vi "Burn-In Testing.vi"() -> ()   [LabVIEW 2012]
uses:
  TestData/Command.ctl
  Controls/Command_Enum.ctl
  Controls/Exit.vi
  Controls/MainRef.ctl
  Controls/Waferimage.ctl
  Controls/TestData.ctl
  Controls/UserInput.ctl
  Controls/MeasureControl.ctl
  Controls/TestArea.ctl
  Controls/WaferDataDisplay.ctl
  Controls/MapPOS.ctl
panel:
  in  "Stop":bool
  in  "Input":T1
  in  "Calibration Wl":dbl
  in  "Wl min,nm":dbl
  in  "Wl max,nm":dbl
  in  "GPIB":string
  in  "Integration Time":i32
  in  "Stop Current,mA":dbl
  in  "Start Current,mA":dbl
  in  "Voltage Compliance,V":dbl
  in  "QuickTest_Display":T2 {"TestData"."50mA Data"."Current,mA" format="%_6g"; "TestData"."50mA Data"."WL" format="%_6g"; "TestData"."50mA Data"."Voltage" format="%_6g"; "TestData"."50mA Data"."Power" format="%_6g"; "TestData"."20mA Data"."Reverse" format="%#_3g"; "TestData"."20mA Data"."Current,mA" format="%_6g"; "TestData"."20mA Data"."Knee Current" format="%#_3g"; "TestData"."20mA Data"."WL" format="%_6g"; "TestData"."20mA Data"."Voltage" format="%_6g"; "TestData"."20mA Data"."Power" format="%_5g"}
  in  "System Back Button":bool
  in  "MapPOS":T5={"Top"={"left"=208, "top"=106, "right"=218, "bottom"=116}, "CenterC"={"left"=217, "top"=189, "right"=228, "bottom"=200}, "CenterB"={"left"=217, "top"=208, "right"=228, "bottom"=219}, "CenterA"={"left"=199, "top"=208, "right"=209, "bottom"=219}, "Left"={"left"=103, "top"=199, "right"=114, "bottom"=209}, "Right"={"left"=314, "top"=199, "right"=325, "bottom"=209}}
  in  "Wafer Data":T6
  out "Wafer":T7
  # "Current Result"
  # "Measure Control"
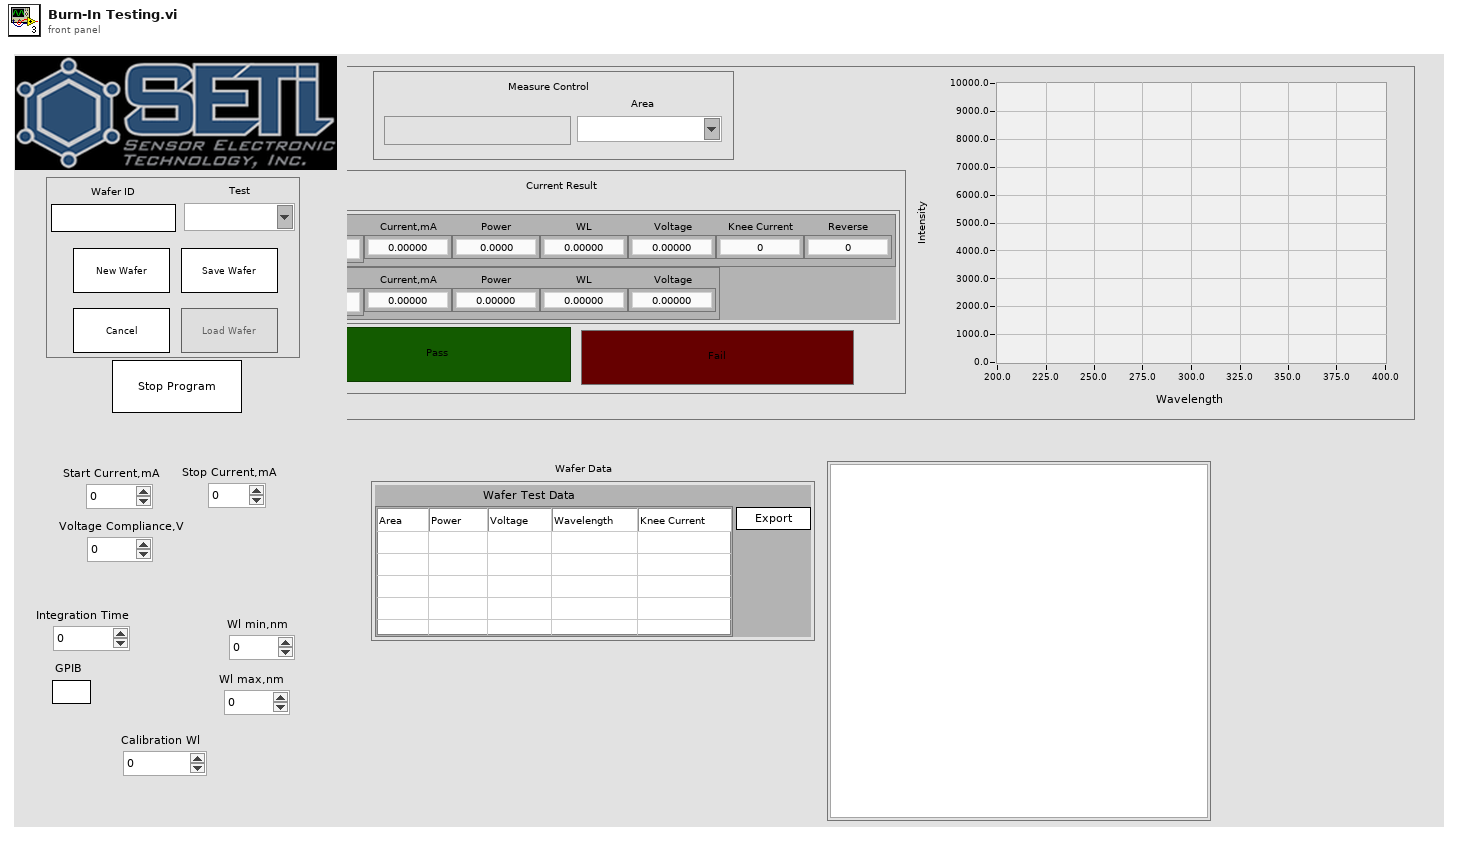
[diagram p1: front panel]
types:
  T1 = typedef "UserInput.ctl" = cluster{"Wafer ID":string, "Test":string, "New":bool, "Save":bool, "Load":bool, "Cancel":bool}
  T2 = typedef "MeasureControl.ctl" = cluster{"Pass":bool, "Fail":bool, "Measure":bool, "Area":T3, "TestData":T4, "Graph":cluster{"Y":dbl[], "Y":dbl[]}[]}
  T3 = typedef "TestArea.ctl" = string
  T4 = typedef "TestData.ctl" = cluster{"20mA Data":cluster{"Area":string, "Current,mA":dbl, "Power":dbl, "WL":dbl, "Voltage":dbl, "Knee Current":dbl, "Reverse":dbl}, "50mA Data":cluster{"Area":string, "Current,mA":dbl, "Power":dbl, "WL":dbl, "Voltage":dbl}}
  T5 = typedef "MapPOS.ctl" = cluster{"Top":cluster{"left":i16, "top":i16, "right":i16, "bottom":i16}, "CenterC":cluster{"left":i16, "top":i16, "right":i16, "bottom":i16}, "CenterB":cluster{"left":i16, "top":i16, "right":i16, "bottom":i16}, "CenterA":cluster{"left":i16, "top":i16, "right":i16, "bottom":i16}, "Left":cluster{"left":i16, "top":i16, "right":i16, "bottom":i16}, "Right":cluster{"left":i16, "top":i16, "right":i16, "bottom":i16}}
  T6 = typedef "WaferDataDisplay.ctl" = cluster{"Wafer Test Data":string[][], "Export":bool}
  T7 = typedef "Waferimage.ctl" = picture
  T8 = typedef "MainRef.ctl" = cluster{"Wafer Data":refnum<vi>, "MeasureCntrl":refnum<vi>, "Input":refnum<vi>, "Wafer":refnum<vi>, "MapPOS":refnum<vi>, "INSTR_PARAM 2":refnum<vi>}
  T9 = typedef "Command.ctl" = cluster{"Command":T10, "Data":variant, "type":variant}
  T10 = typedef "Command_Enum.ctl" = enum16{"INIT", "LOAD", "MEASURE", "NEW", "SAVE", "SWAP_MODE", "UPDATE_ACQ", "EXIT", "CANCEL"}
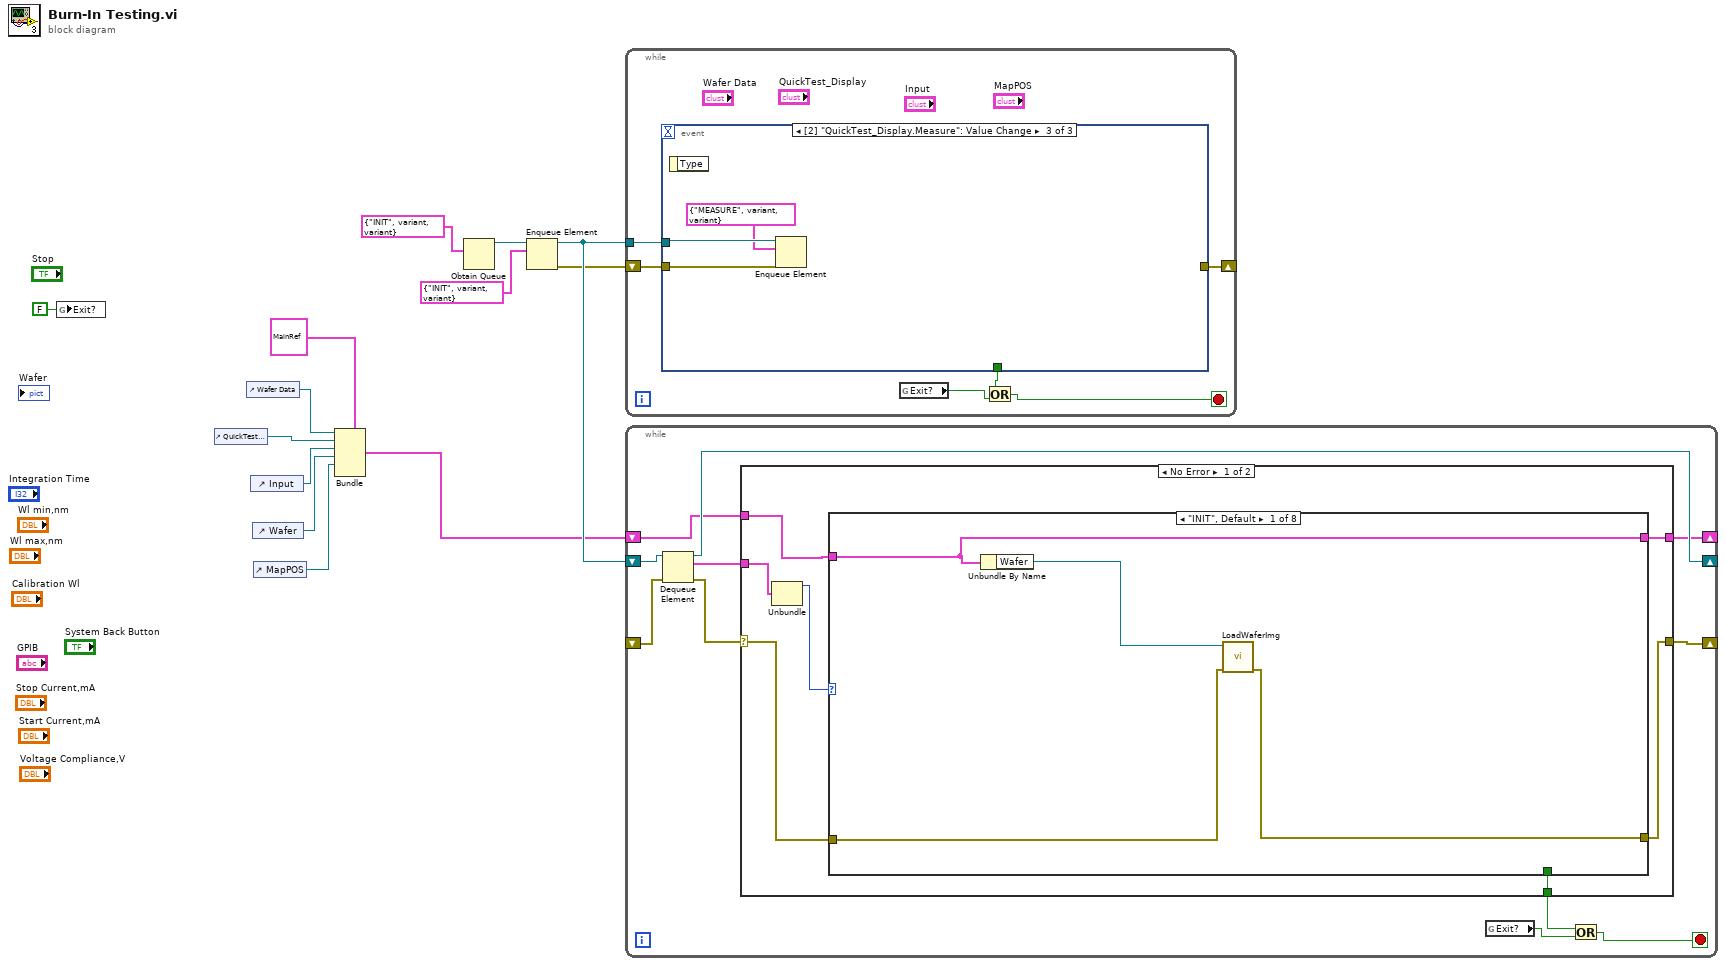
[diagram p0: block diagram]
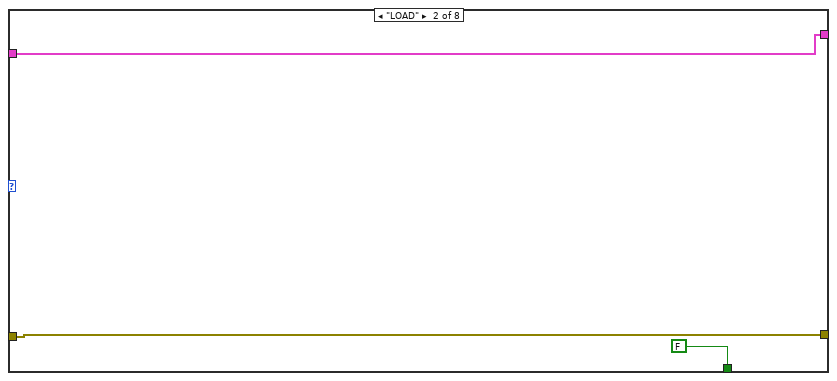
[diagram p2: hidden frame]
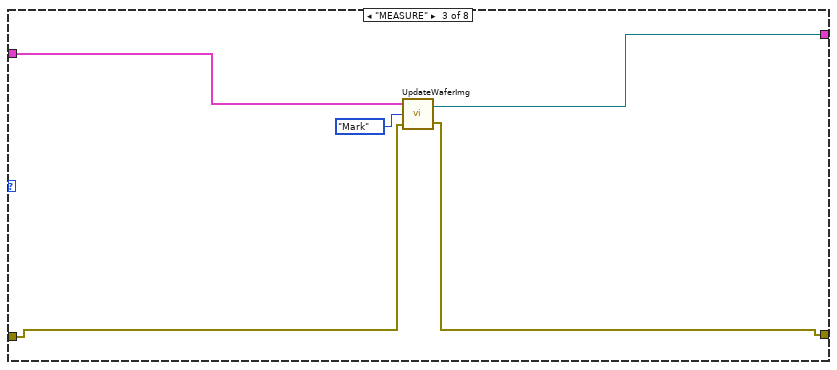
[diagram p3: hidden frame]
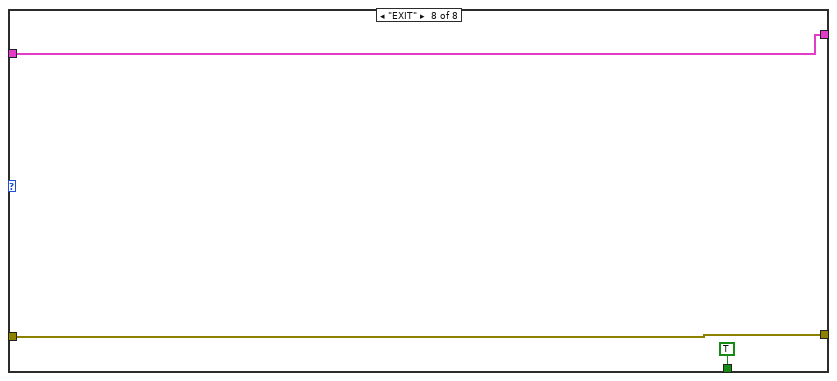
[diagram p8: hidden frame]
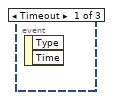
[diagram p10: hidden frame]
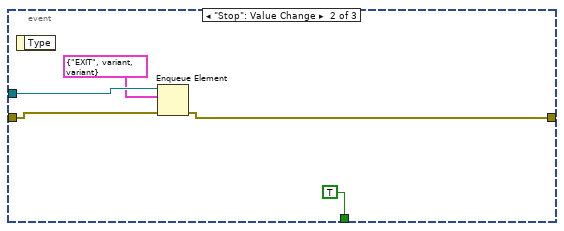
[diagram p11: hidden frame]
diagram:
  n1 = global write "Exit.vi" "Exit?"(FALSE ("Exit?")) -> ()
  n2 = control-ref of="QuickTest_Display"() -> (w6:refnum<vi>)
  n3 = control-ref of="Wafer Data"() -> (w7:refnum<vi>)
  n4 = control-ref of="Input"() -> (w5:refnum<vi>)
  n5 = control-ref of="Wafer"() -> (w4:refnum<vi>)
  n6 = control-ref of="MapPOS"() -> (w2:refnum<vi>)
  n7 = Bundle(cluster=T8 {"Wafer Data"=refnum, "MeasureCntrl"=refnum, "Input"=refnum, "Wafer"=refnum, "MapPOS"=refnum, "INSTR_PARAM 2"=refnum}, "Wafer Data"=w7, "MeasureCntrl"=w6, "Input"=w5, "Wafer"=w4, "MapPOS"=w2) -> (w3:T8)  [unwired: 1 in]
  n8 = Obtain Queue(element data type=T9 {"Command"=enum."INIT", "Data"=variant, "type"=variant} ("Cluster")) -> (queue out=w12:refnum<queue>)  [unwired: 4 in, 2 out]
  n9 = Enqueue Element(queue=w12, element=T9 {"Command"=enum."INIT", "Data"=variant, "type"=variant}) -> (queue out=w10:refnum<queue>, error out=w9:errorcluster)  [unwired: 2 in, 1 out]
  n10 = while {
    tunnel: w10 -> [w19]
    shift-right: [w14] -> _
    shift-left: w9 -> [w15]
    stop <- w17 stop-if-true
    n11 = event shown="[2] \"QuickTest_Display.Measure\": Value Change" {
      selector: _ -> [_ _ _]
      dyn-events: _ -> [_ _ _]
      timeout: _ -> [_ _ _]
      tunnel: w19 -> [_ w23 w27]
      tunnel: [_ TRUE ("x") _] -> w16
      tunnel: w15 -> [_ w21 w26]
      tunnel: [_ w20 _] -> w14
      event Timeout {
        n12 = event-data() -> ()  [unwired: 1 in, 2 out]
      }
      event "Stop": Value Change {
        n13 = event-data() -> ()  [unwired: 1 in, 1 out]
        n14 = Enqueue Element(queue=w23, element=T9 {"Command"=enum."EXIT", "Data"=variant, "type"=variant}, error in (no error)=w21) -> (error out=w20:errorcluster)  [unwired: 1 in, 2 out]
      }
      event Value Change {
        n15 = event-data() -> ()  [unwired: 1 in, 1 out]
        n16 = Enqueue Element(queue=w27, element=T9 {"Command"=enum."MEASURE", "Data"=variant, "type"=variant}, error in (no error)=w26) -> ()  [unwired: 1 in, 3 out]
      }
    }
    n17 = global read "Exit.vi" "Exit?"() -> (w18:bool)
    n18 = Or(x=w16, y=w18) -> (x .or. y?=w17:bool)
  }
  n19 = while {
    shift-right: [w34] -> _
    shift-left: w10 -> [w38]
    shift-right: [w35] -> _
    shift-left: _ -> [w36]
    shift-right: [w28] -> _
    shift-left: w3 -> [w29]
    stop <- w31 stop-if-true
    n20 = Dequeue Element(queue=w38, error in (no error)=w36) -> (queue out=w34:refnum<queue>, element=w33:T9, error out=w37:errorcluster)  [unwired: 1 in, 1 out]
    n21 = case shown="No Error" w37 {
      selector: w37 -> [w41 w70]
      tunnel: [w42 w70] -> w35
      tunnel: w33 -> [w45 _]
      tunnel: [w43 _] -> w30
      tunnel: w29 -> [w40 w69]
      tunnel: [w39 w69] -> w28
      frame No Error {
        n22 = Unbundle(w45) -> ("Command"=w44:T10)  [unwired: 2 out]
        n23 = case shown="\"INIT\", Default" w44 {
          tunnel: [_ FALSE ("y") _ _ _ _ _ TRUE ("y")] -> w43
          tunnel: [w46 w51 w54 w59 w61 w63 w65 w67] -> w42
          tunnel: w41 -> [w49 w51 w53 w59 w61 w63 w65 w67]
          tunnel: w40 -> [w48 w50 w56 w58 w60 w62 w64 w66]
          tunnel: [w48 w50 w55 w58 w60 w62 w64 w66] -> w39
          frame "INIT", Default {
            n24 = Unbundle By Name(w48) -> ("Wafer"=w47:refnum<vi>)
            n25 = call "LoadWaferImg.vi"("error in (no error)"=w49, "FrontPanelData.lvclass"=w47) -> ("error out"=w46:errorcluster)  [unwired: 8 in, 1 out]
          }
          frame "LOAD" {
          }
          frame "MEASURE" {
            n26 = call "UpdateWaferImg.vi"("error in (no error)"=w53, "Enum"=enum16{"Mark", "Clear All"}."Mark", "Wrapper In"=w56) -> ("error out"=w54:errorcluster, "Wrapper Out"=w55:refnum<class "EpiWrapper.lvclass">)
          }
          frame "NEW" {
          }
          frame "SAVE" {
          }
          frame "SWAP_MODE" {
          }
          frame "UPDATE_ACQ" {
          }
          frame "EXIT" {
          }
        }
      }
      frame Error {
      }
    }
    n27 = global read "Exit.vi" "Exit?"() -> (w32:bool)
    n28 = Or(x=w30, y=w32) -> (x .or. y?=w31:bool)
  }
